vi "Speed Global.vi"() -> ()   [LabVIEW 2013]
panel:
  out "Speed (RPM)":fxp<+/-,28,17>[](array[numeric])
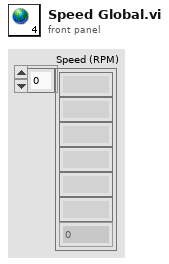
[diagram p1: front panel]
diagram:
